vi "Global - Pressure Data.vi"() -> ()   [LabVIEW 2019]
uses:
  Data.ctl
panel:
  in  "Data":T1
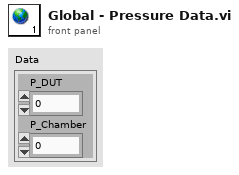
[diagram p1: front panel]
types:
  T1 = typedef "Data.ctl" = cluster{"P_DUT":dbl, "P_Chamber":dbl}
diagram:
